vi "Quaternion Interpolation.vi"(2 "end pose":T1=[[0.2818556107229001, -0.49341675968208987, -0.8228592321708784, 0.11697004227643469], [-0.7778734424176673, -0.6195744782940995, 0.10507318129704712, 0.030499600323496263], [-0.5616674481268332, 0.6104648778688426, -0.5584463363683838, -0.2863453905069739], [0.0, 0.0, 0.0, 1.0]] format="%#_2g", 3 "intermediate points":i32=10, 4 "start pose":T1=[[1.0, 0.0, 0.0, 0.0], [0.0, 1.0, 0.0, 0.0], [0.0, 0.0, 1.0, 0.0], [0.0, 0.0, 0.0, 1.0]]) -> (1 "interpolations":dbl[][][](array[numeric]))   [LabVIEW 2024]
uses:
  <vilib>/Analysis/Matrix/Datatypes/RealMatrix.ctl
  <vilib>/Analysis/Matrix/NI_Matrix.lvlib
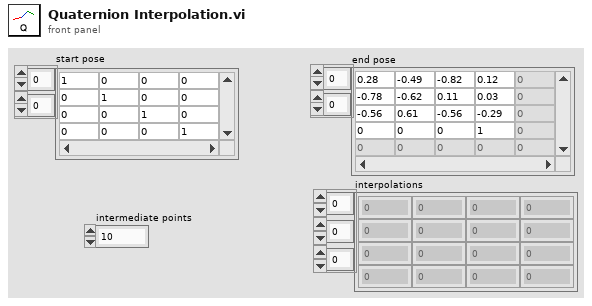
[diagram p1: front panel]
types:
  T1 = typedef "NI_Matrix.lvlib/RealMatrix.ctl" = dbl[][]
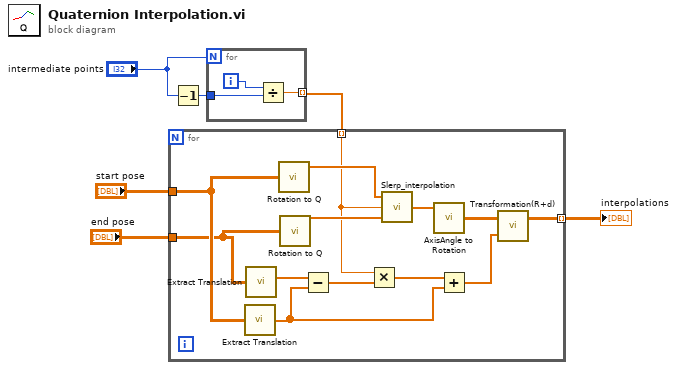
[diagram p0: block diagram]
diagram:
  n1 = Decrement(x="intermediate points") -> (x-1=w4:i32)
  n2 = for {
    N: "intermediate points" -> [_]
    tunnel: w4 -> [w9]
    tunnel: [w7] -> w2 mode=indexing
    i -> [w8]
    n3 = Divide(x=w8, y=w9) -> (x/y=w7:dbl)
  }
  n4 = for {
    tunnel: [w14] -> w1 mode=indexing
    tunnel: "start pose" -> [w18]
    tunnel: "end pose" -> [w17]
    tunnel: w2 -> [w11] mode=indexing
    n5 = call <userlib>:"Extract Translation.vi"("Transformation matrix"=w18) -> ("Position"=w19:dbl[])
    n6 = call <userlib>:"Extract Translation.vi"("Transformation matrix"=w17) -> ("Position"=w20:dbl[])
    n7 = call <userlib>:"Rotation to Q.vi"("Rotation matrix"=w18) -> ("quaternion"=w13:dbl[])  [unwired: 2 out]
    n8 = call <userlib>:"Rotation to Q.vi"("Rotation matrix"=w17) -> ("quaternion"=w12:dbl[])  [unwired: 2 out]
    n9 = Subtract(x=w20, y=w19) -> (x-y=w21:dbl[])
    n10 = Multiply(x=w11, y=w21) -> (x*y=w22:dbl[])
    n11 = call <userlib>:"Slerp_interpolation.vi"("quaternion 2"=w12, "ratio"=w11, "quaternion 1"=w13) -> ("interpolated quaternion"=w10:dbl[])  [unwired: 2 in]
    n12 = call <userlib>:"AxisAngle to Rotation.vi"("quaternion"=w10) -> ("rotation matrix"=w16:T1)  [unwired: 2 in]
    n13 = Add(x=w22, y=w19) -> (x+y=w15:dbl[])
    n14 = call <userlib>:"Transformation(R+d).vi"("Translation"=w15, "rotation matrix"=w16) -> ("Transformation matrix"=w14:T1)  [unwired: 1 in]
  }
  "interpolations" <- w1
